vi "Create Log File Path.vi"(8 "error in (no error)":errorcluster) -> (0 "error out":errorcluster, 3 "dup path":path)   [LabVIEW 2025]
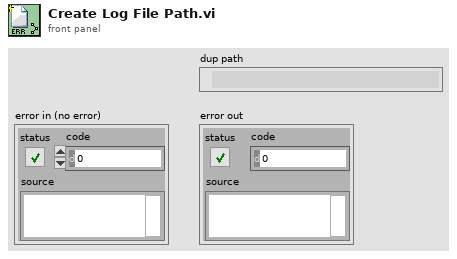
[diagram p1: front panel]
types:
  T1 = enum16{"open", "replace", "create", "open or create", "replace or create", "replace or create with confirmation"}
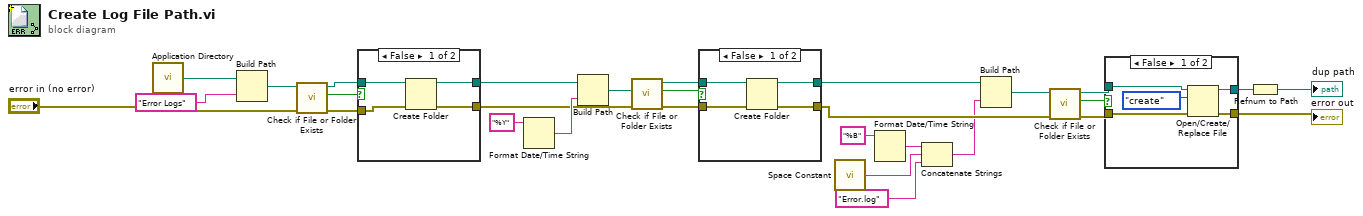
[diagram p0: block diagram]
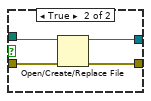
[diagram p2: hidden frame]
diagram:
  n1 = call <vilib>:"Application Directory.vi"() -> ("Application Directory"=w2:path)
  n2 = Build Path(base path=w2, name or relative path="Error Logs") -> (appended path=w4:path)
  n3 = call <vilib>:"Check if File or Folder Exists.vi"("error in (no error)"="error in (no error)", "path"=w4) -> ("error out"=w7:errorcluster, "file or folder exists?"=w5:bool, "dup path"=w6:path)  [unwired: 7 in]
  n4 = case shown="False" w5 {
    tunnel: w6 -> [w33 w35]
    tunnel: w7 -> [w32 w34]
    tunnel: [w31 w35] -> w12
    tunnel: [w30 w34] -> w8
    frame False {
      n5 = Create Folder(path (use dialog)=w33, error in=w32) -> (created path=w31:path, error out=w30:errorcluster)  [unwired: 1 in, 1 out]
    }
    frame True {
    }
  }
  n6 = Format Date/Time String(time format string (%c)="%Y") -> (date/time string=w15:string)  [unwired: 2 in]
  n7 = Build Path(base path=w12, name or relative path=w15) -> (appended path=w13:path)
  n8 = call <vilib>:"Check if File or Folder Exists.vi"("error in (no error)"=w8, "path"=w13) -> ("error out"=w11:errorcluster, "file or folder exists?"=w10:bool, "dup path"=w9:path)  [unwired: 7 in]
  n9 = case shown="False" w10 {
    tunnel: w9 -> [w39 w41]
    tunnel: w11 -> [w38 w40]
    tunnel: [w37 w41] -> w16
    tunnel: [w36 w40] -> w23
    frame False {
      n10 = Create Folder(path (use dialog)=w39, error in=w38) -> (created path=w37:path, error out=w36:errorcluster)  [unwired: 1 in, 1 out]
    }
    frame True {
    }
  }
  n11 = call <vilib>:"Space Constant.vi"() -> ("String"=w20:string)
  n12 = Format Date/Time String(time format string (%c)="%B") -> (date/time string=w18:string)  [unwired: 2 in]
  n13 = Concatenate Strings(w18, w20, "Error.log" ("string")) -> (w21:string)
  n14 = Build Path(base path=w16, name or relative path=w21) -> (appended path=w22:path)
  n15 = call <vilib>:"Check if File or Folder Exists.vi"("error in (no error)"=w23, "path"=w22) -> ("error out"=w26:errorcluster, "file or folder exists?"=w25:bool, "dup path"=w24:path)  [unwired: 7 in]
  n16 = case shown="False" w25 {
    tunnel: w24 -> [w46 w47]
    tunnel: w26 -> [w45 w50]
    tunnel: [w44 w48] -> w27
    tunnel: [w43 w49] -> w28
    frame False {
      n17 = Open/Create/Replace File(file path (use dialog)=w46, error in=w45, operation (0:open)=T1."create") -> (refnum out=w44:refnum<file>, error out=w43:errorcluster)  [unwired: 3 in, 1 out]
    }
    frame True {
      n18 = Open/Create/Replace File(file path (use dialog)=w47, error in=w50) -> (refnum out=w48:refnum<file>, error out=w49:errorcluster)  [unwired: 4 in, 1 out]
    }
  }
  "error out" <- w28
  n19 = Refnum to Path(1:w27) -> (0:→"dup path":path)
